vi "HP 3325B Function Gen.vi"(1 "stop":ext=10000000.0 format="%.3f", 2 "start":ext=1000000.0 format="%.3f", 3 "sweep function (none:0)":u16(ring) items=["no sweep", "linear single", "linear cont.", "log single", "log cont."], 4 "phase (deg)":ext format="%.2f", 5 "GPIB address":i32, 6 "sweep time (S)":ext=1.0 format="%.2f", 8 "frequency (Hz)":ext=1000.0 format="%.3f", 9 "offset (V)":ext format="%.2f", 10 "amplitude (V)":ext=1.0 format="%.4f", 11 "signal type (dc:0)":u16(ring) items=["dc ", "sine", "square", "triangle", "pos. ramp", "neg. ramp"]) -> ()   [LabVIEW 2018]
panel:
  out "full command string":string
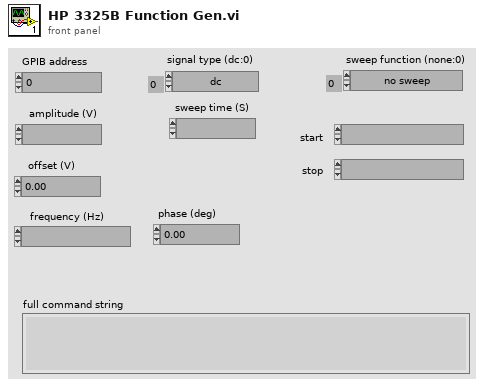
[diagram p1: front panel]
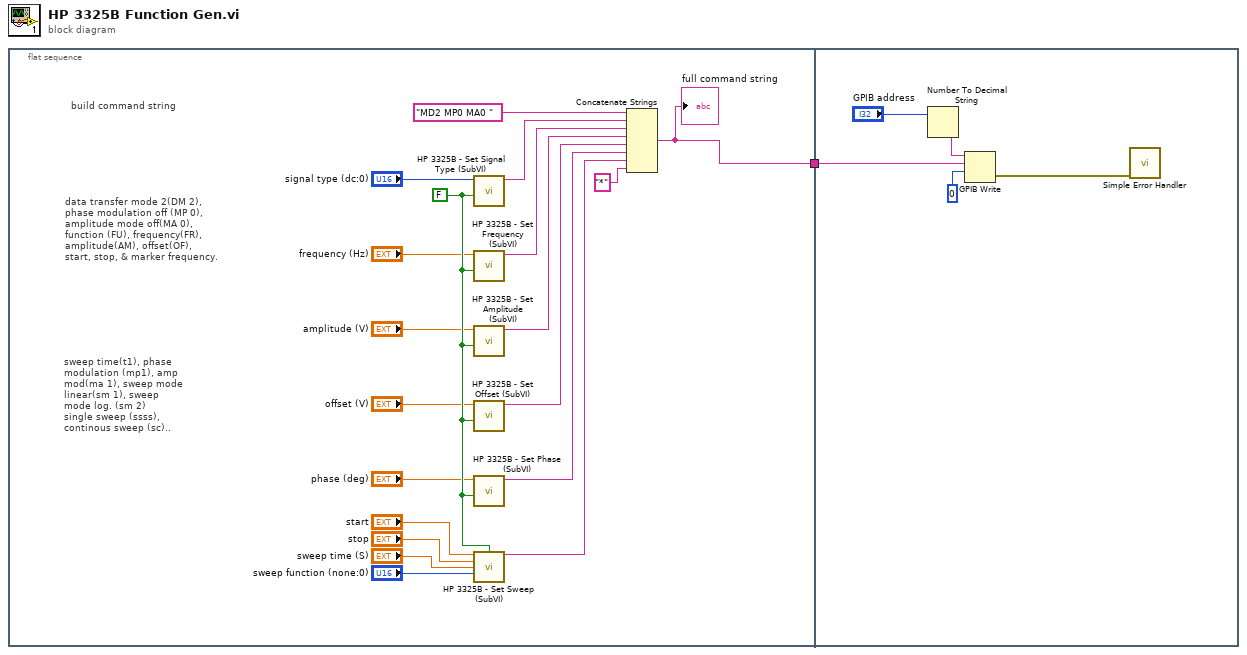
[diagram p0: block diagram]
diagram:
  n1 = flat-sequence {
    tunnel: [w2] -> w1
    tunnel: w1 -> [w21]
    frame #0 {
      w19 = FALSE
      # "sweep time(t1), phase\nmodulation (mp1), amp\nmod(ma 1), sweep mode\nlinear(sm 1), sweep \nmode log. (sm 2)\nsingle sweep (ssss),\ncontinous sweep (sc).."
      # "data transfer mode 2(DM 2),\nphase modulation off (MP 0),\namplitude mode off(MA 0),\nfunction (FU), frequency(FR),\namplitude(AM), offset(OF),\nstart, stop, & marker frequency."
      # "build command string"
      n2 = call "HP 3325B - Set Signal Type (SubVI).vi"("write?"=w19, "signal type (dc:0)"="signal type (dc:0)") -> ("command string"=w9:string)  [unwired: 8 in, 1 out]
      n3 = call "HP 3325B - Set Frequency (SubVI).vi"("write?"=w19, "frequency (Hz)"="frequency (Hz)") -> ("command string"=w8:string)  [unwired: 8 in, 1 out]
      n4 = call "HP 3325B - Set Amplitude (SubVI).vi"("write?"=w19, "amplitude (V)"="amplitude (V)") -> ("command string"=w7:string)  [unwired: 8 in, 1 out]
      n5 = call "HP 3325B - Set Offset (SubVI).vi"("write?"=w19, "offset (V)"="offset (V)") -> ("command string"=w6:string)  [unwired: 8 in, 1 out]
      n6 = call "HP 3325B - Set Phase (SubVI).vi"("write?"=w19, "phase (deg)"="phase (deg)") -> ("command string"=w5:string)  [unwired: 8 in, 1 out]
      n7 = call "HP 3325B - Set Sweep (SubVI).vi"("start"="start", "write?"=w19, "stop"="stop", "sweep time (s)"="sweep time (S)", "sweep function (none:0)"="sweep function (none:0)") -> ("command string"=w4:string)  [unwired: 9 in, 1 out]
      n8 = Concatenate Strings("MD2 MP0 MA0 ", w9, w8, w7, w6, w5, w4, "*") -> (w2:string)
      "full command string" <- w2
    }
    frame #1 {
      n9 = Number To Decimal String(number="GPIB address") -> (decimal integer string=w23:string)  [unwired: 1 in]
      n10 = GPIB Write(0:w23, 1:w21, 2:0) -> (6:w22:errorcluster)  [unwired: 1 in, 2 out]
      n11 = call <vilib>:"Simple Error Handler.vi"("error in (no error)"=w22) -> ()  [unwired: 4 in, 5 out]
    }
  }
